vi "Test Drive OO.vi"() -> ()   [LabVIEW 2016]
uses:
  Ocean optics configuration.ctl
  Utilities/Fit/Multi-peak Parameters.ctl
  Utilities/Fit/Peak Parameters.ctl
  Ocean Optics Driver.lvclass
  C:/github/NHMFL_Core/Libraries/Instruments/VISA Instrument/VISA Instrument.lvclass
  VISA Instrument/VISA Instrument.lvclass/VISA Instrument.ctl
  VISA Instrument/Write VISA resource.vi
  Write Ocean optics configuration.vi
panel:
  in  "VISA resource name":refnum<visa-resource-name>="MayaPro"
  out "Spectral Waveform":T1(graph)
  in  "Ocean optics configuration":T2={"Integration time"=0.5, "Fit parameters"={"Peaks"=[{"Amplitude"=4000.0, "Center"=694.3, "Width"=0.4}, {"Amplitude"=2000.0, "Center"=692.8, "Width"=0.4}], "Slope"=0.0, "Intercept"=0.0, "Function"=enum."Gauss"}, "Fit"=FALSE, "Use last fit as  guess"=FALSE, "Window width"=690.0, "Repeat"=3, "Reference wavelengh"=694.123} {"Integration time" format="%#_6ps"}
  in  "Device":string="MayaPro"
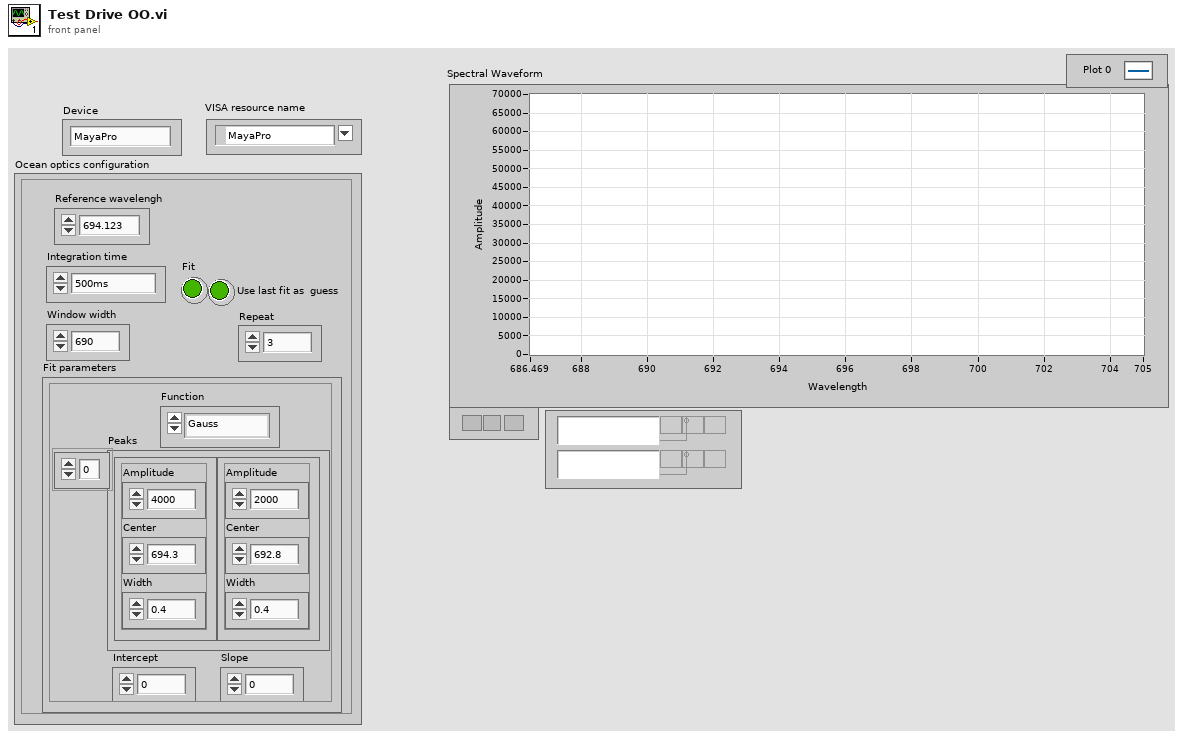
[diagram p1: front panel]
types:
  T1 = cluster{"Wavelength (nm)":dbl[], "Spectrum by Pixel Number":dbl[]}[]
  T2 = typedef "Ocean optics configuration.ctl" = cluster{"Integration time":dbl, "Fit parameters":T3, "Fit":bool, "Use last fit as  guess":bool, "Window width":dbl, "Repeat":i32, "Reference wavelengh":dbl}
  T3 = typedef "Multi-peak Parameters.ctl" = cluster{"Peaks":T4[], "Slope":dbl, "Intercept":dbl, "Function":enum16{"Gauss", "Lorentz"}}
  T4 = typedef "Peak Parameters.ctl" = cluster{"Amplitude":dbl, "Center":dbl, "Width":dbl}
  T5 = cluster{"Wavelengths":dbl[], "Spectrum by Pixel Number":dbl[]}[]
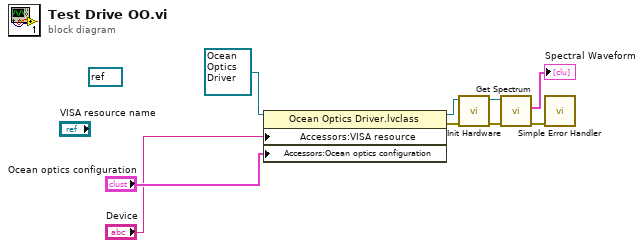
[diagram p0: block diagram]
diagram:
  (unwired) refnum<visa-resource-name> refnum ("VISA resource")
  n1 = property class="Ocean Optics Driver.lvclass"(reference=refnum<class "Ocean Optics Driver.lvclass"> refnum ("Ocean Optics Driver.lvclass"), "Accessors:VISA resource"="Device", "Accessors:Ocean optics configuration"="Ocean optics configuration") -> (reference out=w8:refnum<class "Ocean Optics Driver.lvclass">, error out=w7:errorcluster)  [unwired: 1 in]
  n2 = call-dynamic "Init Hardware.vi"("error in (no error)"=w7, "Ocean Optics Driver in"=w8) -> ("error out"=w4:errorcluster, "Ocean Optics Driver out"=w5:refnum<class "Ocean Optics Driver.lvclass">)  [unwired: 8 in]
  n3 = call-dynamic "Get Spectrum.vi"("error in (no error)"=w4, "Ocean Optics Driver in"=w5) -> ("error out"=w2:errorcluster, "Spectrum Graph"=→"Spectral Waveform":T5)  [unwired: 7 in, 1 out]
  n4 = call <vilib>:"Simple Error Handler.vi"("error in (no error)"=w2) -> ()  [unwired: 4 in, 5 out]
